vi "Add Channel.vi"(7 "Type":T1, 8 "error in (no error)":errorcluster, 10 "Channel Name":string, 11 "User BluelinesRedlines in":refnum<class "User BluelinesRedlines.lvclass">) -> (0 "error out":errorcluster, 3 "User BluelinesRedlines out":refnum<class "User BluelinesRedlines.lvclass">)   [LabVIEW 2020, in "VolatusGUIElements.lvlib" / "User BluelinesRedlines.lvclass"]
uses:
  User BluelinesRedlines.lvclass
  User BluelinesRedlines.lvclass/User BluelinesRedlines.ctl
  VolatusGUI/BluelinesRedlines Source/Range Limit Config.ctl
  VolatusGUI/BluelinesRedlines Source/BluelinesRedlines Source.lvclass
  VolatusGUI/BluelinesRedlines Source/BLRL Type.ctl
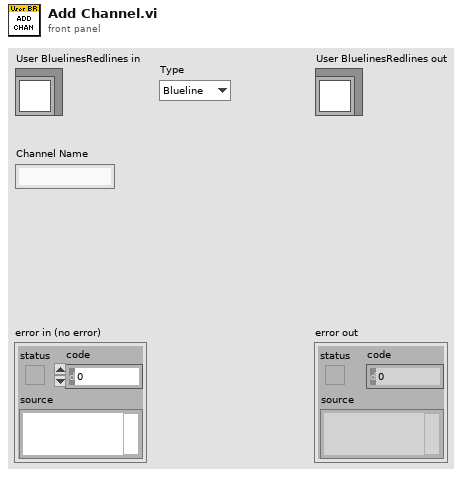
[diagram p1: front panel]
types:
  T1 = typedef "VolatusGUI.lvlib/BluelinesRedlines Source.lvclass/BLRL Type.ctl" = enum16{"Blueline", "Redline"}
  T2 = typedef "VolatusGUI.lvlib/BluelinesRedlines Source.lvclass/Range Limit Config.ctl" = cluster{"Channel":string, "Low Limit":dbl, "High Limit":dbl}
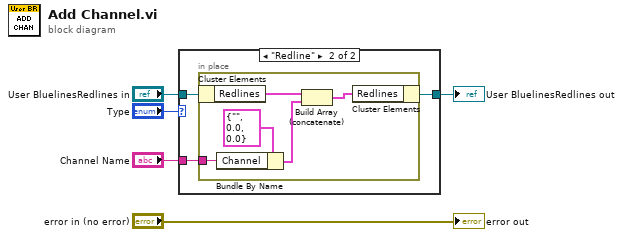
[diagram p0: block diagram]
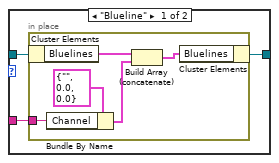
[diagram p2: hidden frame]
diagram:
  n1 = case shown="\"Redline\"" "Type" {
    tunnel: "User BluelinesRedlines in" -> [w8 w16]
    tunnel: "Channel Name" -> [w7 w15]
    tunnel: [w6 w14] -> w1
    frame "Blueline" {
      n2 = in-place {
        in-place-border: w7 -> [w12]
        n3 = in-place-cluster #1(w8) -> ("Bluelines"=w11:T2[])
        n4 = Bundle By Name(cluster=T2 {"Channel"="", "Low Limit"=0.0, "High Limit"=0.0} ("Range Limit Config"), "Channel"=w12) -> (w10:T2)
        n5 = Build Array (concatenate)(w11, w10) -> (w9:T2[])
        n6 = in-place-cluster #1("Bluelines"=w9) -> (w6:refnum<class "User BluelinesRedlines.lvclass">)
      }
    }
    frame "Redline" {
      n7 = in-place {
        in-place-border: w15 -> [w20]
        n8 = in-place-cluster #2(w16) -> ("Redlines"=w19:T2[])
        n9 = Bundle By Name(cluster=T2 {"Channel"="", "Low Limit"=0.0, "High Limit"=0.0} ("Range Limit Config"), "Channel"=w20) -> (w18:T2)
        n10 = Build Array (concatenate)(w19, w18) -> (w17:T2[])
        n11 = in-place-cluster #2("Redlines"=w17) -> (w14:refnum<class "User BluelinesRedlines.lvclass">)
      }
    }
  }
  "User BluelinesRedlines out" <- w1
  "error out" <- "error in (no error)"
